vi "ShowExtrapolationResults.vi"(8 "error in (no error)":errorcluster, 10 "Analysis in":refnum<class "Analysis.lvclass">, 11 "Table Control":refnum<vi>) -> (0 "error out":errorcluster, 2 "Analysis out":refnum<class "Analysis.lvclass">)   [LabVIEW 2015]
doc: "Loads the Extrapolation Results from the AnalysisObject and displays the data in the Table"
uses:
  MSControl/Classes/Analysis/Analysis.lvclass
  <vilib>/Utility/miscctls.llb/LVRowAndColumnUnsignedTypeDef.ctl
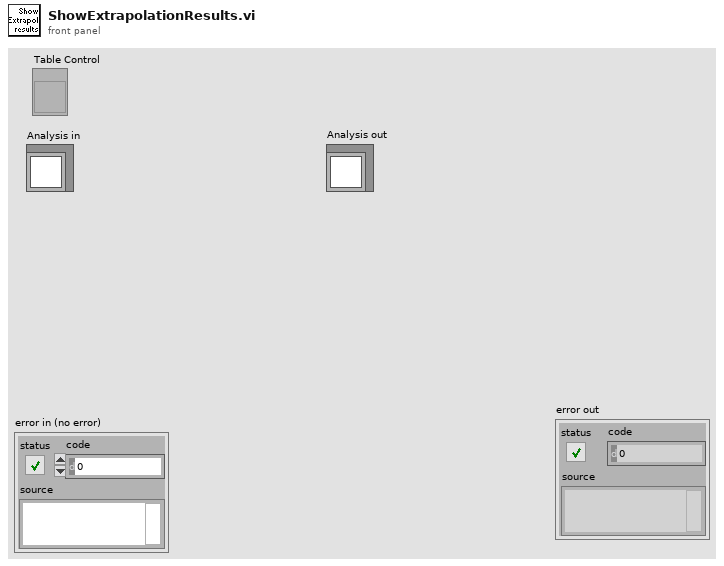
[diagram p1: front panel]
types:
  T1 = typedef "LVRowAndColumnUnsignedTypeDef.ctl" = cluster{"Row":u32, "Column":u32}
  T2 = typedef "ExtrapolationResultsArray.ctl" = string[][]
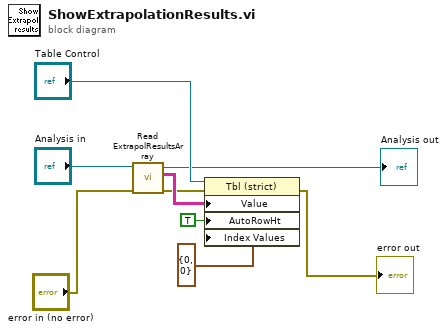
[diagram p0: block diagram]
diagram:
  n1 = call-dynamic "Read ExtrapolResultsArray.vi"("error in (no error)"="error in (no error)", "Analysis in"="Analysis in") -> ("error out"=w4:errorcluster, "ExtrapolResultsArray"=w6:T2, "Analysis out"=→"Analysis out":refnum<class "Analysis.lvclass">)  [unwired: 7 in]
  n2 = property class="Tbl (strict)"(reference="Table Control", error in=w4, "Value"=w6, "AutoRowHt"=TRUE ("Autosizing Row Height"), "Index Values"=T1 {"Row"=0, "Column"=0}) -> (error out=→"error out":errorcluster)  [unwired: 1 out]
